vi "mtg reader - collect session folders.vi"(7 "action":enum16{"init", "refresh", "select one"}(ring), 8 "error in (no error)":errorcluster, 10 "selected folder":string=" ", 11 "config":T1={"path calling vi"=path "", "base directory"="data (sessions)", "session folders table"=refnum}) -> (0 "error out":errorcluster, 3 "selected session folder":path)   [LabVIEW 2025]
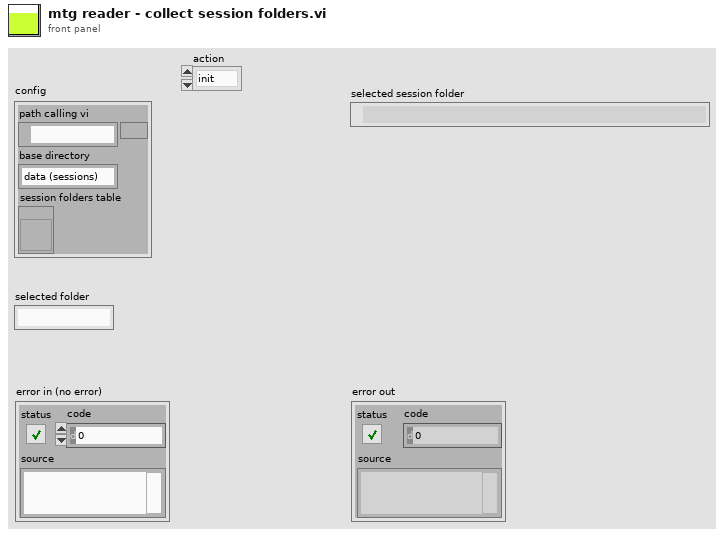
[diagram p1: front panel]
types:
  T1 = cluster{"path calling vi":path, "base directory":string, "session folders table":refnum<vi>}
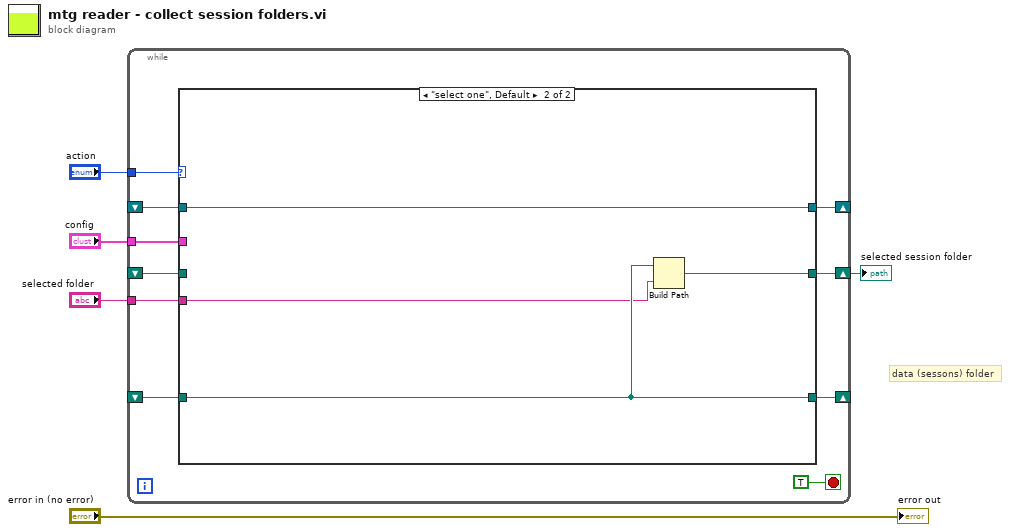
[diagram p0: block diagram]
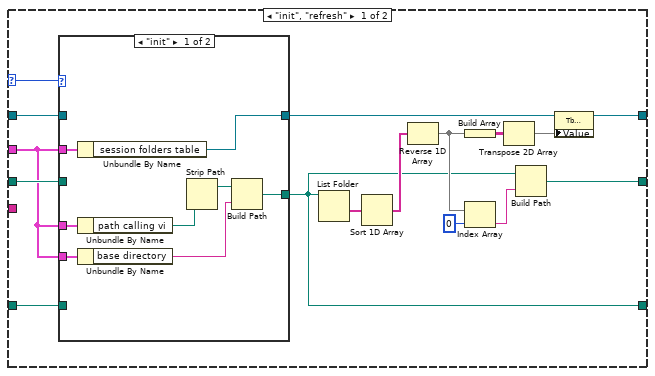
[diagram p2: hidden frame]
diagram:
  # "data (sessons) folder"
  n1 = while {
    shift-right: [w15] -> w5
    shift-left: _ -> [w13]
    tunnel: "action" -> [w14]
    shift-right: [w12] -> _
    shift-left: _ -> [w11]
    shift-right: [w10] -> _
    shift-left: _ -> [w9]
    tunnel: "config" -> [w7]
    tunnel: "selected folder" -> [w6]
    stop <- TRUE stop-if-true
    n2 = case shown="\"select one\", Default" w14 {
      selector: w14 -> [w21 _]
      tunnel: [w29 w44] -> w15
      tunnel: w13 -> [w18 _]
      tunnel: [w25 w45] -> w12
      tunnel: w11 -> [w19 w45]
      tunnel: [w22 w43] -> w10
      tunnel: w9 -> [w17 w43]
      tunnel: w7 -> [w16 _]
      tunnel: w6 -> [_ w42]
      frame "init", "refresh" {
        n3 = case shown="\"init\"" w21 {
          tunnel: [w38 w40] -> w22
          tunnel: [w36 w41] -> w20
          tunnel: w19 -> [_ w41]
          tunnel: w18 -> [_ _]
          tunnel: w17 -> [_ w40]
          tunnel: w16 -> [w37 _]
          tunnel: w16 -> [w35 _]
          tunnel: w16 -> [w33 _]
          frame "init" {
            n4 = Unbundle By Name(w37) -> ("session folders table"=w36:refnum<vi>)
            n5 = Unbundle By Name(w33) -> ("path calling vi"=w32:path)
            n6 = Unbundle By Name(w35) -> ("base directory"=w34:string)
            n7 = Strip Path(path=w32) -> (stripped path=w39:path)  [unwired: 1 out]
            n8 = Build Path(base path=w39, name or relative path=w34) -> (appended path=w38:path)
          }
          frame "refresh", Default {
          }
        }
        n9 = List Folder(path=w22) -> (folder names=w27:string[])  [unwired: 3 in, 3 out]
        n10 = Sort 1D Array(array=w27) -> (sorted array=w30:string[])
        n11 = Reverse 1D Array(array=w30) -> (reversed array=w24:string[])
        n12 = Build Array(w24) -> (w31:string[][])
        n13 = Index Array(array=w24, index=0) -> (element=w28:string)
        n14 = Transpose 2D Array(2D array=w31) -> (transposed array=w26:string[][])
        n15 = Build Path(base path=w22, name or relative path=w28) -> (appended path=w29:path)
        n16 = property class="Tbl (strict)"(reference=w20, "Value"=w26) -> (reference out=w25:refnum<vi>)  [unwired: 1 in, 1 out]
      }
      frame "select one", Default {
        n17 = Build Path(base path=w43, name or relative path=w42) -> (appended path=w44:path)
      }
    }
  }
  "selected session folder" <- w5
  "error out" <- "error in (no error)"
